vi "Get items.vi"(8 "error in (no error)":errorcluster, 11 "MsgPackArray in":refnum<class "MsgPackArray.lvclass">) -> (0 "error out":errorcluster, 2 "Bytes":u8[](array[numeric]), 3 "MsgPackArray out":refnum<class "MsgPackArray.lvclass">)   [LabVIEW 2020, in "MessagePack.lvlib" / "MsgPackArray.lvclass"]
uses:
  MsgPackArray.lvclass
  MsgPackArray.lvclass/MsgPackArray.ctl
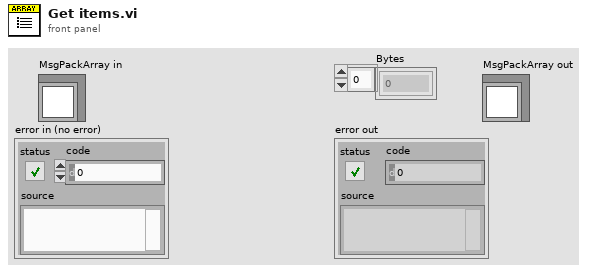
[diagram p1: front panel]
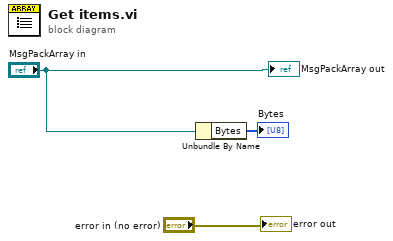
[diagram p0: block diagram]
diagram:
  n1 = Unbundle By Name("MsgPackArray in") -> ("Bytes"=→"Bytes":u8[])
  "MsgPackArray out" <- "MsgPackArray in"
  "error out" <- "error in (no error)"
